vi "CS-4 Revision Query.vi"(8 "error in (no error)":errorcluster, 11 "VISA session":refnum<visa-resource-name>) -> (0 "error out":errorcluster, 1 "Instr Firmware Revision":string, 2 "Instr Driver Revision":string, 3 "dup VISA session":refnum<visa-resource-name>)   [LabVIEW 2016]
doc: "This VI queries the current instrument firmware revision and instrument driver revision.\n\nThis Instrument Driver's Revision number is 1.0 and is compatable with Instrument Firmware Revision 1.xx\n\n(CS-4)\nCreated By: Wayne Holloway\nRelease Date: 5/05/99\nOriginally Developed in LabVIEW Version: 4.1\n\nModification History: \n\nNone"
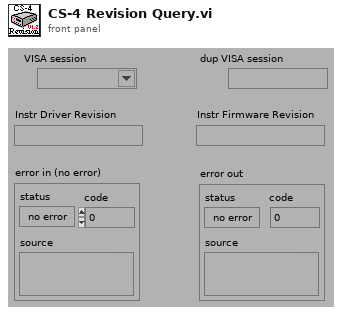
[diagram p1: front panel]
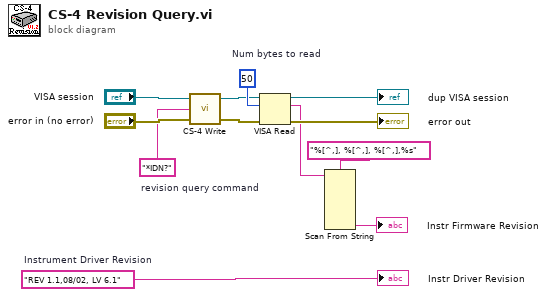
[diagram p0: block diagram]
diagram:
  w5 = "*IDN?"  # revision query command
  w3 = u32 50  # Num bytes to read
  w12 = "REV 1.1,08/02, LV 6.1"  # Instrument Driver Revision
  n1 = call "CS-4 Write.vi"("error in (no error)"="error in (no error)", "write buffer (\"\")"=w5, "VISA session"="VISA session") -> ("error out"=w4:errorcluster, "dup VISA session"=w2:refnum<visa-resource-name>)  [unwired: 1 out]
  n2 = VISA Read(VISA resource name=w2, byte count=w3, error in (no error)=w4) -> (VISA resource name out=→"dup VISA session":refnum<visa-resource-name>, read buffer=w6:string, error out=→"error out":errorcluster)  [unwired: 1 out]
  n3 = Scan From String(format string="%[^,], %[^,], %[^,],%s", input string=w6) -> (output 4=→"Instr Firmware Revision":string)  [unwired: 9 in, 3 out]
  "Instr Driver Revision" <- w12
